vi "channel.list.vi"(8 "error in":errorcluster, 10 "data source rid":string, 11 "Client in":refnum<class "Client.lvclass">) -> (0 "error out":errorcluster, 2 "List":refnum<class "List.lvclass">, 3 "Client out":refnum<class "Client.lvclass">)   [LabVIEW 2020, in "Client.lvclass"]
doc: "Lists all channels available on a given dataset, video, or connection."
uses:
  Client.lvclass
  Client.lvclass/Client.ctl
  client.lvlib
  List/List.lvclass
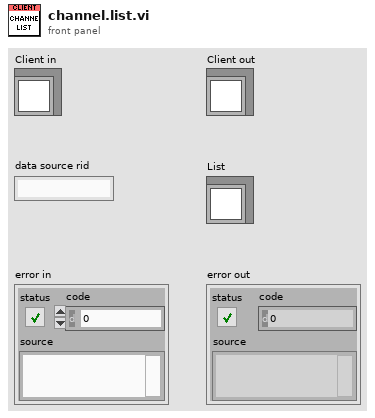
[diagram p1: front panel]
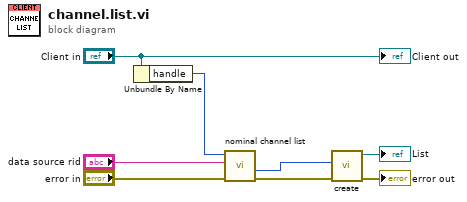
[diagram p0: block diagram]
diagram:
  n1 = Unbundle By Name("Client in") -> ("handle"=w7:i32)
  n2 = call "nominal channel list.vi"("error in (no error)"="error in", "data_source_rid"="data source rid", "client"=w7) -> ("error out"=w3:errorcluster, "out_list out"=w4:i32)  [unwired: 5 in, 2 out]
  n3 = call "create.vi"("error in (no error)"=w3, "handle"=w4) -> ("error out"=→"error out":errorcluster, "List out"=→"List":refnum<class "List.lvclass">)  [unwired: 8 in]
  "Client out" <- "Client in"
